vi "DrawTopics.vi"(2 "Selection":i32) -> (3 "new picture":picture, 4 "Status":string, 5 "all good?":bool, 6 "Boundaries":cluster{i32, i32}[](array[cluster])=[{10, 22}, {30, 42}, {50, 62}])   [LabVIEW 2012]
uses:
  <vilib>/Utility/miscctls.llb/LVRectTypeDef.ctl
  MyState.ctl
panel:
  out "Status":T1[](array[typedef])
  out "Servers":string[](array[string])
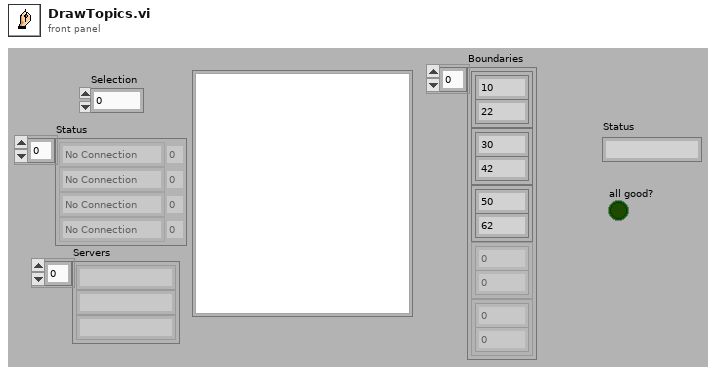
[diagram p1: front panel]
types:
  T1 = typedef "MyState.ctl" = enum16{"No Connection", "Registered", "Connected", "Close"}
  T2 = enum16{"Add Server", "Clear Server", "Clear All", "Get Info", "GetPanelInfo"}
  T3 = cluster{"left":i16, "top":i16, "right":i16, "bottom":i16}
  T4 = typedef "LVRectTypeDef.ctl" = cluster{"Left":i16, "Top":i16, "Right":i16, "Bottom":i16}
  T5 = typedef "imagedata.ctl" = cluster{"image type":i32, "image depth":i32, "image":u8[], "mask":u8[], "colors":u32[], "Rectangle":cluster{"left":i16, "top":i16, "right":i16, "bottom":i16}}
  T6 = cluster{"horizontal":enum16{"left", "center", "right"}, "vertical":enum16{"top", "center", "bottom"}}
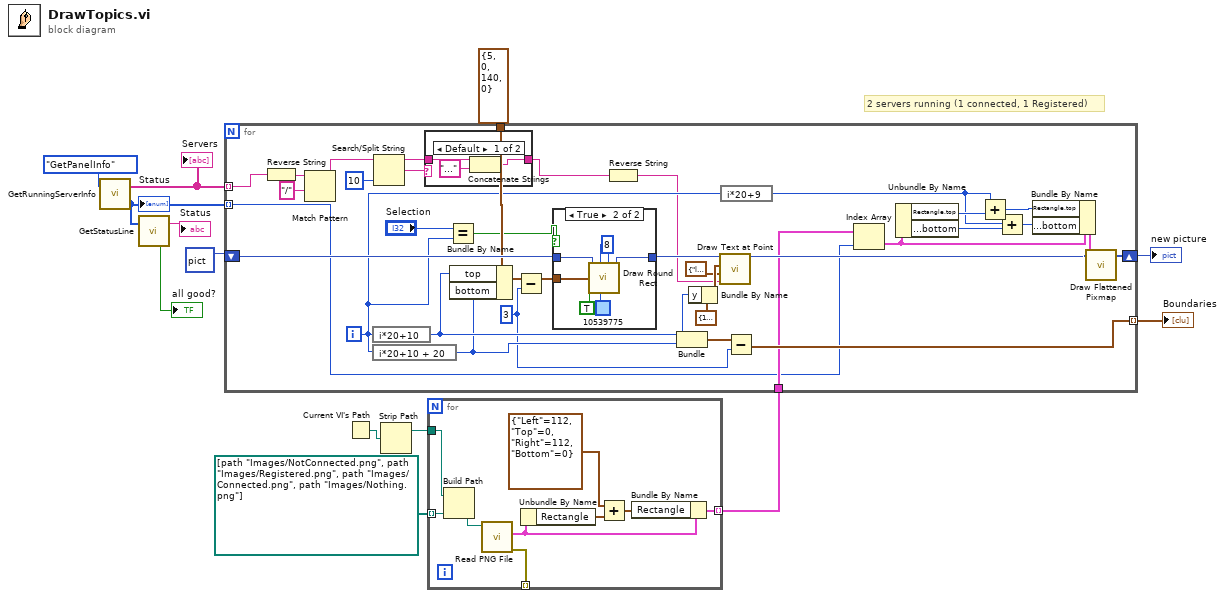
[diagram p0: block diagram]
diagram:
  # "2 servers running (1 connected, 1 Registered)"
  n1 = call "GetRunningServerInfo.vi"("Task"=T2."GetPanelInfo") -> ("Status"=w4:T1[], "Topics"=w5:string[])  [unwired: 1 in, 1 out]
  "Servers" <- w5
  "Status" <- w4
  n2 = call "GetStatusLine.vi"("Status"=w4) -> ("all good?"=→"all good?":bool, "Status"=→"Status":string)  [unwired: 1 in]
  n3 = Current VI's Path() -> (path=w8:path)
  n4 = Strip Path(path=w8) -> (stripped path=w7:path)  [unwired: 1 out]
  n5 = for {
    tunnel: [w20] -> w9 mode=indexing
    tunnel: w7 -> [w17]
    tunnel: path[] [path "Images/NotConnected.png", path "Images/Registered.png", path "Images/Connected.png", path "Images/Nothing.png"] -> [w16] mode=indexing
    tunnel: [w14] -> _ mode=indexing
    n6 = Build Path(base path=w17, name or relative path=w16) -> (appended path=w15:path)
    n7 = call <vilib>:"Read PNG File.vi"("path to PNG file"=w15) -> ("error out"=w14:errorcluster, "image data"=w21:T5)  [unwired: 8 in, 1 out]
    n8 = Unbundle By Name(w21) -> ("Rectangle"=w19:T3)
    n9 = Add(x=T4 {"Left"=112, "Top"=0, "Right"=112, "Bottom"=0} ("Bounds"), y=w19) -> (x+y=w18:T4)
    n10 = Bundle By Name(cluster=w21, "Rectangle"=w18) -> (w20:T5)
  }
  n11 = for {
    tunnel: w5 -> [w31] mode=indexing
    shift-right: [w43] -> w13
    shift-left: picture data[5B] ("new picture") -> [w54]
    tunnel: [w49] -> w11 mode=indexing
    tunnel: T3 {"left"=5, "top"=0, "right"=140, "bottom"=0} ("rect") -> [w50]
    tunnel: w9 -> [w41]
    tunnel: w4 -> [w32] mode=indexing
    i -> [w36]
    w46 = i16 3 ("oval width")
    n12 = Reverse String(1:w31) -> (0:w30:string)
    n13 = Match Pattern(string=w30, regular expression="/") -> (before substring=w27:string)  [unwired: 1 in, 3 out]
    n14 = expression code="i*20+10"(w36) -> (w52:i32)
    n15 = expression code="i*20+10 + 20"(w36) -> (w51:i32)
    n16 = Search/Split String(string=w27, offset (0)=10) -> (substring before match=w23:string, match + rest of string=w25:string)  [unwired: 1 in, 1 out]
    n17 = case shown="Default" w25 {
      tunnel: [w61 w62] -> w24
      tunnel: w23 -> [w60 w62]
      frame Default {
        n18 = Concatenate Strings(w60, "..." ("string")) -> (w61:string)
      }
      frame "" {
      }
    }
    n19 = Equal?(x="Selection", y=w36) -> (x = y?=w44:bool)
    n20 = Bundle By Name(cluster=w50, "top"=w52, "bottom"=w51) -> (w48:T3)
    n21 = Subtract(x=w48, y=w46) -> (x-y=w47:T3)
    n22 = case shown="True" w44 {
      tunnel: w54 -> [w63 w66]
      tunnel: [w63 w65] -> w53
      tunnel: w47 -> [_ w64]
      frame False {
      }
      frame True {
        w67 = i16 8 ("oval width")
        n23 = call <vilib>:"Draw Round Rect.vi"("picture"=w66, "oval width"=w67, "rect"=w64, "fill?(F)"=TRUE, "color(black)"=u32 10539775, "oval height"=w67) -> ("new picture"=w65:picture)  [unwired: 3 in]
      }
    }
    n24 = Reverse String(1:w24) -> (0:w28:string)
    n25 = Bundle(w52, w51) -> (w56:cluster{i32, i32})  [unwired: 1 in]
    n26 = Bundle By Name(cluster=cluster{"x":i16, "y":i16} {"x"=10, "y"=0} ("origin"), "y"=w52) -> (w57:cluster{"x":i16, "y":i16})
    n27 = call <vilib>:"Draw Text at Point.vi"("text"=w28, "alignment(left, top)"=T6 {"horizontal"=enum."left", "vertical"=enum."top"}, "origin"=w57, "picture"=w53) -> ("new picture"=w42:picture)  [unwired: 6 in, 1 out]
    n28 = expression code="i*20+9"(w36) -> (w34:i32)
    n29 = Subtract(x=w56, y=w46) -> (x-y=w49:cluster{i32, i32})
    n30 = Index Array(array=w41, index=w32) -> (element=w37:T5)
    n31 = Unbundle By Name(w37) -> ("Rectangle.top"=w39:i16, "Rectangle.bottom"=w35:i16)
    n32 = Add(x=w34, y=w39) -> (x+y=w40:i32)
    n33 = Add(x=w35, y=w34) -> (x+y=w33:i32)
    n34 = Bundle By Name(cluster=w37, "Rectangle.top"=w40, "Rectangle.bottom"=w33) -> (w38:T5)
    n35 = call <vilib>:"Draw Flattened Pixmap.vi"("image data"=w38, "picture"=w42) -> ("new picture"=w43:picture)  [unwired: 7 in]
  }
  "new picture" <- w13
  "Boundaries" <- w11
